vi "Solenoid - 3WAY.vi"(8 "Error In":errorcluster, 10 "OPEN CLOSE":enum8{"TANK", "DRAIN"}(ring), 11 "VISA session":refnum<visa-resource-name>="MW100") -> (0 "Error Out":errorcluster, 3 "dup VISA session":refnum<visa-resource-name>)   [LabVIEW 2009]
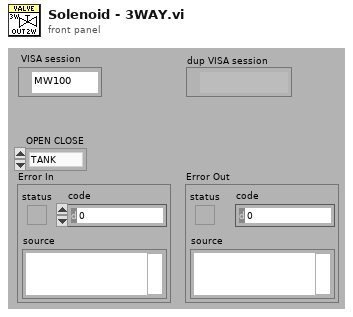
[diagram p1: front panel]
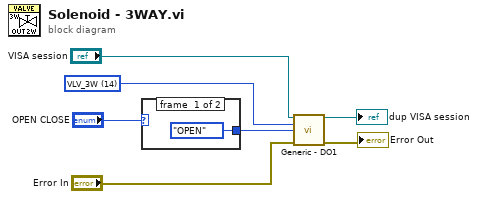
[diagram p0: block diagram]
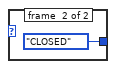
[diagram p2: hidden frame]
diagram:
  w2 = u16 14 items=["RTD_IN", "RTD_OUT", "RTD_AMB", "Tc_1", "Tc_2", "Tc_3", "Tc_4", "Tc_5", "Tc_6", "Tc_down", "Pres_HI1", "Pres_HI2", "Pres_LOW", "VLV_IN", "VLV_3W", "VLV_OUT", "PWR_MAIN", "FLOWMETER", "4-20_OUT", "HEATER_TOP", "HEATER_BOT", "COMPRESSOR", "DRM_LOW", "DRM_HIGH", "INTF_TEMPFLO", "INTF_READY", "INTF_START", "INTF_STOP"] ("Channel_Enum")
  n1 = case shown="\"DRAIN\"" "OPEN CLOSE" {
    tunnel: [enum8{"CLOSED", "OPEN"}."OPEN" ("Relay Status (0:CLOSED)") enum8{"CLOSED", "OPEN"}."CLOSED" ("Relay Status (0:CLOSED)")] -> w3
    frame #0 {
    }
    frame #1 {
    }
  }
  n2 = call "Generic - DO1.vi"("VISA session"="VISA session", "Channel_Enum"=w2, "Relay Status (0:CLOSED)"=w3, "Error In"="Error In") -> ("dup VISA session"=→"dup VISA session":refnum<visa-resource-name>, "error out"=→"Error Out":errorcluster)  [unwired: 10 in]
